vi "Get Unique Log Name.vi"() -> (3 "Log File Name":string)   [LabVIEW 2017, in "TestTextFileSink.lvclass"]
uses:
  TestTextFileSink.lvclass
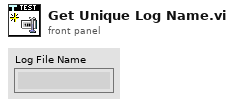
[diagram p1: front panel]
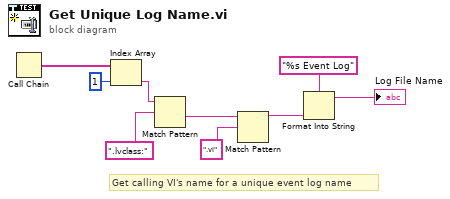
[diagram p0: block diagram]
diagram:
  # "Get calling VI's name for a unique event log name"
  n1 = Call Chain() -> (call chain=w9:string[])
  n2 = Index Array(array=w9, index=1) -> (element=w8:string)
  n3 = Match Pattern(string=w8, regular expression=".lvclass:") -> (after substring=w5:string)  [unwired: 1 in, 3 out]
  n4 = Match Pattern(string=w5, regular expression=".vi") -> (before substring=w3:string)  [unwired: 1 in, 3 out]
  n5 = Format Into String(format string="%s Event Log", w3) -> (resulting string=→"Log File Name":string)  [unwired: 2 in, 1 out]
